vi "UpdatePredecessor.vi"(8 "error in (no error)":errorcluster, 9 "Cost":dbl, 10 "Predecessor Node Ref":refnum<data-value>, 11 "DirectedGraphMapNode in":refnum<class "NI_Robotics_DirectedGraphMapNode.lvclass">) -> (0 "error out":errorcluster, 3 "DirectedGraphMapNode out":refnum<class "NI_Robotics_DirectedGraphMapNode.lvclass">)   [LabVIEW 2017, in "NI_Robotics_DirectedGraphMapNode.lvclass"]
uses:
  <vilib>/robotics/Navigation/shared/MapNode/DirectedGraphMapNode/NI_Robotics_DirectedGraphMapNode.lvclass
  <vilib>/robotics/Navigation/shared/MapNode/AbstractDstarNode/NI_Robotics_AbstractDstarNode.lvclass
  c:/Program Files (x86)/National Instruments/LabVIEW 2017/vi.lib/robotics/Navigation/shared/MapNode/AbstractMapNode/NI_Robotics_AbstractMapNode.lvclass
  <vilib>/robotics/Navigation/shared/MapNode/DirectedGraphMapNode/NI_Robotics_DirectedGraphMapNode.lvclass/NI_Robotics_DirectedGraphMapNode.ctl
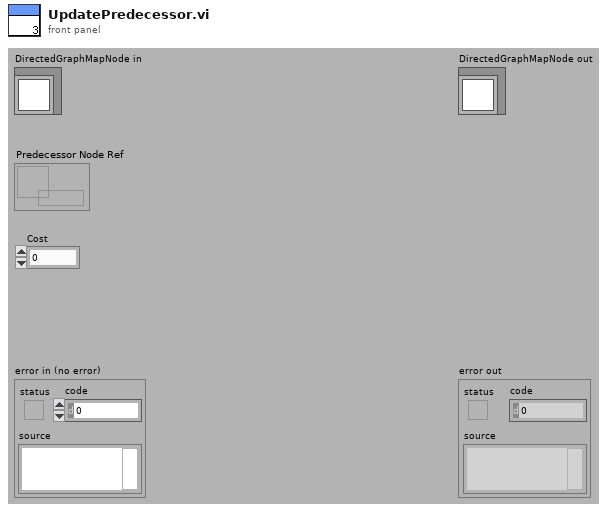
[diagram p1: front panel]
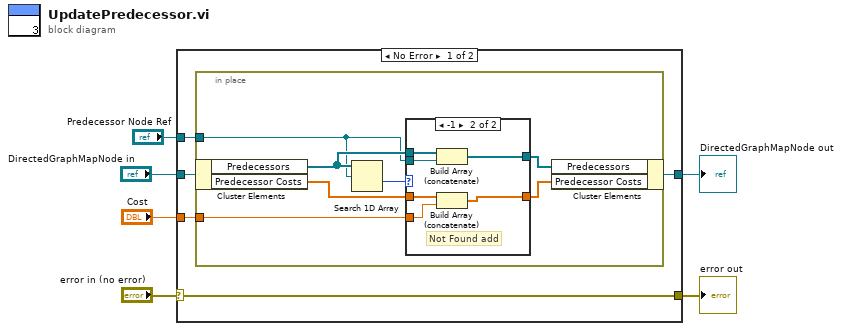
[diagram p0: block diagram]
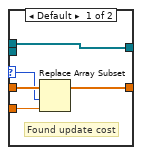
[diagram p2: hidden frame]
diagram:
  n1 = case shown="No Error" "error in (no error)" {
    selector: "error in (no error)" -> [w11 w31]
    tunnel: [w11 w31] -> w5
    tunnel: [w7 w30] -> w3
    tunnel: "DirectedGraphMapNode in" -> [w10 w30]
    tunnel: "Predecessor Node Ref" -> [w9 _]
    tunnel: "Cost" -> [w8 _]
    frame No Error {
      n2 = in-place {
        in-place-border: w9 -> [w16]
        in-place-border: w8 -> [w14]
        n3 = in-place-cluster #1(w10) -> ("Predecessors"=w17:refnum<data-value>[], "Predecessor Costs"=w15:dbl[])
        n4 = Search 1D Array(1D array=w17, element=w16) -> (index of element=w18:i32)  [unwired: 1 in]
        n5 = case shown="-1" w18 {
          selector: w18 -> [w21 _]
          tunnel: w17 -> [w19 w29]
          tunnel: w16 -> [_ w28]
          tunnel: w15 -> [w23 w27]
          tunnel: w14 -> [w22 w26]
          tunnel: [w19 w25] -> w13
          tunnel: [w20 w24] -> w12
          frame Default {
            # "Found update cost"
            n6 = Replace Array Subset(array=w23, new element=w22, index=w21) -> (w20:dbl[])
          }
          frame -1 {
            # "Not Found add"
            n7 = Build Array (concatenate)(w29, w28) -> (w25:refnum<data-value>[])
            n8 = Build Array (concatenate)(w27, w26) -> (w24:dbl[])
          }
        }
        n9 = in-place-cluster #1("Predecessors"=w13, "Predecessor Costs"=w12) -> (w7:refnum<class "NI_Robotics_DirectedGraphMapNode.lvclass">)
      }
    }
    frame Error {
    }
  }
  "error out" <- w5
  "DirectedGraphMapNode out" <- w3
